vi "WS1050 Gen Drivers.vi"(8 "error in (no error)":errorcluster) -> (0 "error out":errorcluster, 3 "WS1050 Drivers":string[](array[string]))   [LabVIEW 2012]
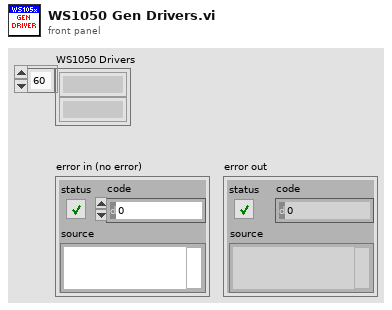
[diagram p1: front panel]
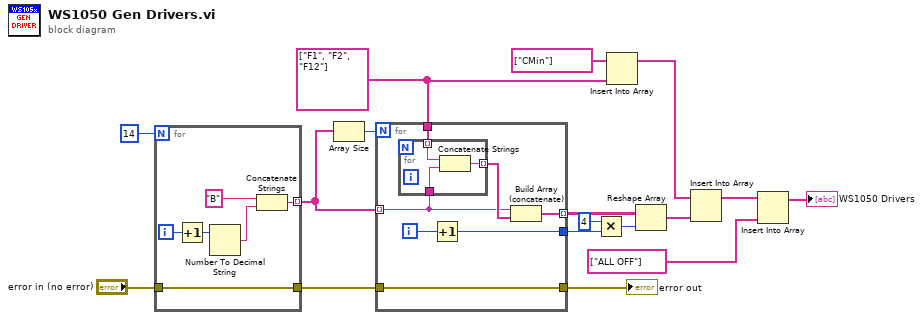
[diagram p0: block diagram]
diagram:
  w2 = string[] ["F1", "F2", "F12"]
  n1 = for {
    N: 14 -> [_]
    tunnel: [w21] -> w15 mode=indexing
    tunnel: "error in (no error)" -> [w19]
    tunnel: [w19] -> w5
    i -> [w20]
    n2 = Increment(x=w20) -> (x+1=w18:i32)
    n3 = Number To Decimal String(number=w18) -> (decimal integer string=w22:string)  [unwired: 1 in]
    n4 = Concatenate Strings("B", w22) -> (w21:string)
  }
  n5 = Array Size(array=w15) -> (size(s)=w16:i32)
  n6 = for {
    N: w16 -> [_]
    tunnel: w15 -> [w25] mode=indexing
    tunnel: w2 -> [w30]
    tunnel: [w26] -> w14 mode=indexing
    tunnel: [w28] -> w12
    tunnel: w5 -> [w24]
    tunnel: [w24] -> w4
    i -> [w29]
    n7 = for {
      tunnel: w25 -> [w32]
      tunnel: w30 -> [w33] mode=indexing
      tunnel: [w31] -> w27 mode=indexing
      n8 = Concatenate Strings(w33, w32) -> (w31:string)
    }
    n9 = Increment(x=w29) -> (x+1=w28:i32)
    n10 = Build Array (concatenate)(w25, w27) -> (w26:string[])
  }
  "error out" <- w4
  n11 = Multiply(x=4, y=w12) -> (x*y=w13:i32)
  n12 = Insert Into Array(array=string[] ["CMin"], new element=w2) -> (w1:string[])  [unwired: 1 in]
  n13 = Reshape Array(w14, w13) -> (w10:string[])
  n14 = Insert Into Array(array=w1, new element=w10) -> (w9:string[])  [unwired: 1 in]
  n15 = Insert Into Array(array=w9, new element=string[] ["ALL OFF"]) -> (→"WS1050 Drivers":string[])  [unwired: 1 in]
